vi "Day06-03_지진 계측기.vi"() -> ()   [LabVIEW 2021]
uses:
  <vilib>/Utility/sysdir.llb/System Directory Type.ctl
  <vilib>/DAQmx/configure/timing.llb/DAQmx Timing (Sample Clock).vi
  <vilib>/DAQmx/create/channels.llb/DAQmx Create Channel (AI-Voltage-Basic).vi
  <vilib>/DAQmx/read.llb/DAQmx Read (Analog Wfm 1Chan NSamp).vi
  <vilib>/numeric/Random Number (Range) U64.vi
panel:
  in  "정지":bool
  in  "파일저장":bool
  in  "알람리셋":bool
  in  "감지시작":bool
  out "알림":bool
  out "출력메시지":string
  out "지진센서값출력":dbl(graph)
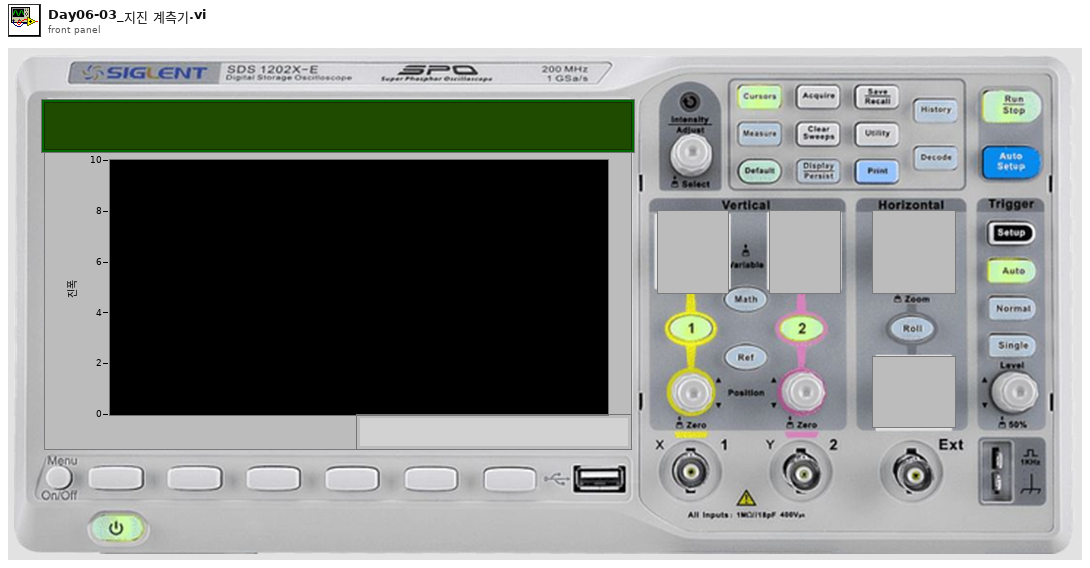
[diagram p1: front panel]
types:
  T1 = typedef "지진 계측기 상태 열거형 상수.ctl" = enum16{"초기화", "대기", "감지 시작", "알림 리셋", "정지"}
  T2 = cluster{"상태":T1, "알림":bool, "출력메시지":string, "지진센서값":dbl, "시간상수":i32}
  T3 = typedef "컨트롤 5.ctl" = enum16{"초기화", "대기", "감지시작", "알람리셋", "정지", "파일저장"}
  T4 = enum16{"open", "replace", "create", "open or create", "replace or create", "replace or create with confirmation"}
  T5 = typedef "System Directory Type.ctl" = i32
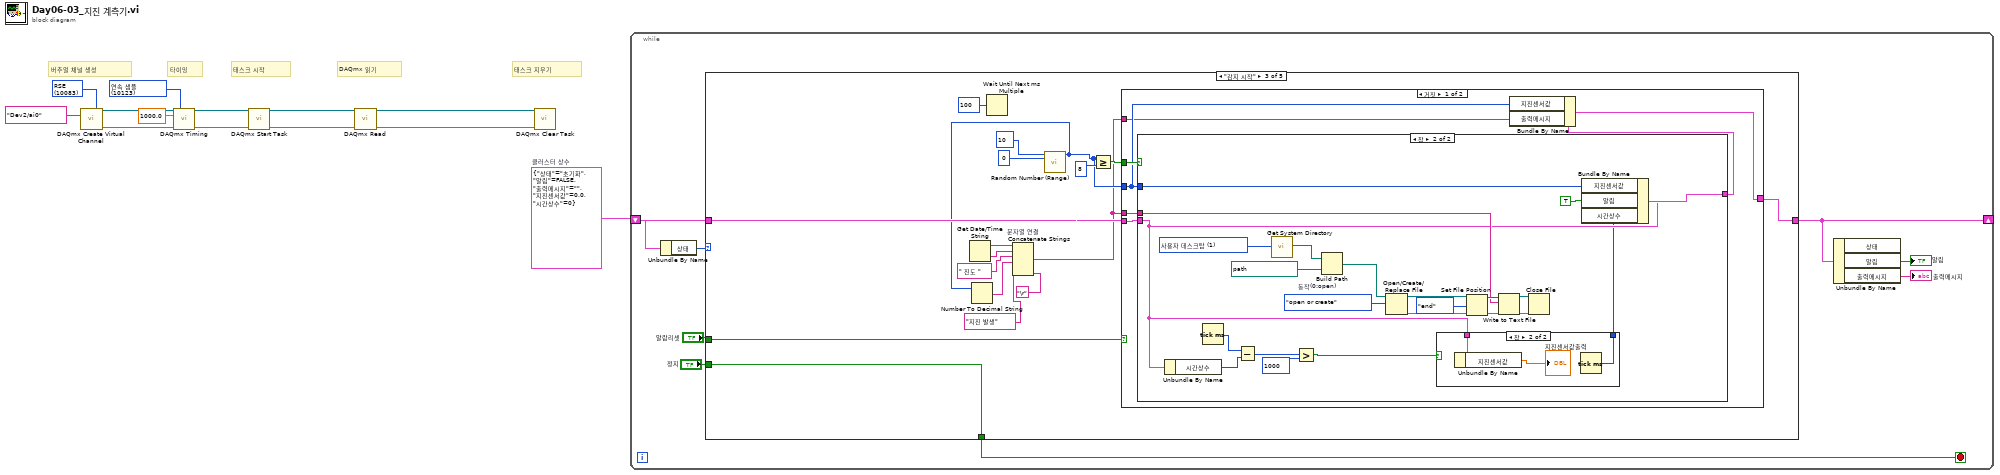
[diagram p0: block diagram]
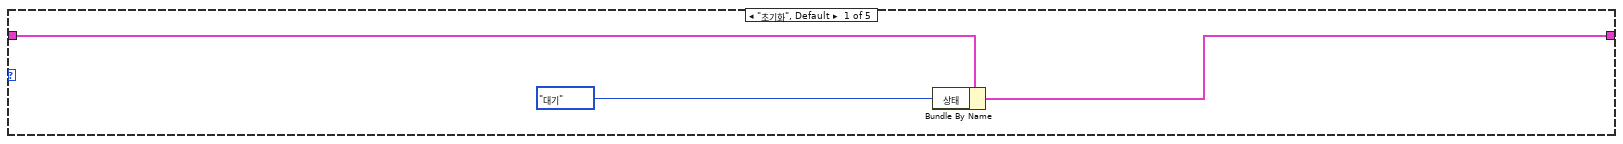
[diagram p2: hidden frame]
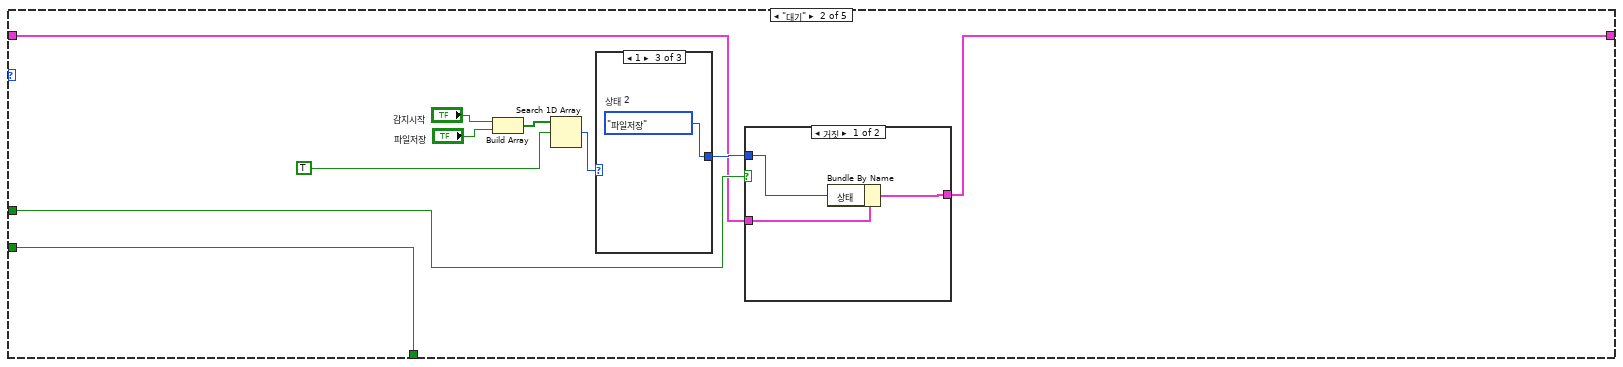
[diagram p3: hidden frame]
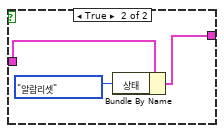
[diagram p4: hidden frame]
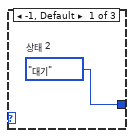
[diagram p5: hidden frame]
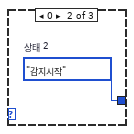
[diagram p6: hidden frame]
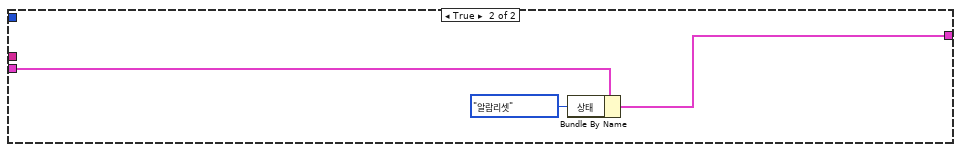
[diagram p9: hidden frame]
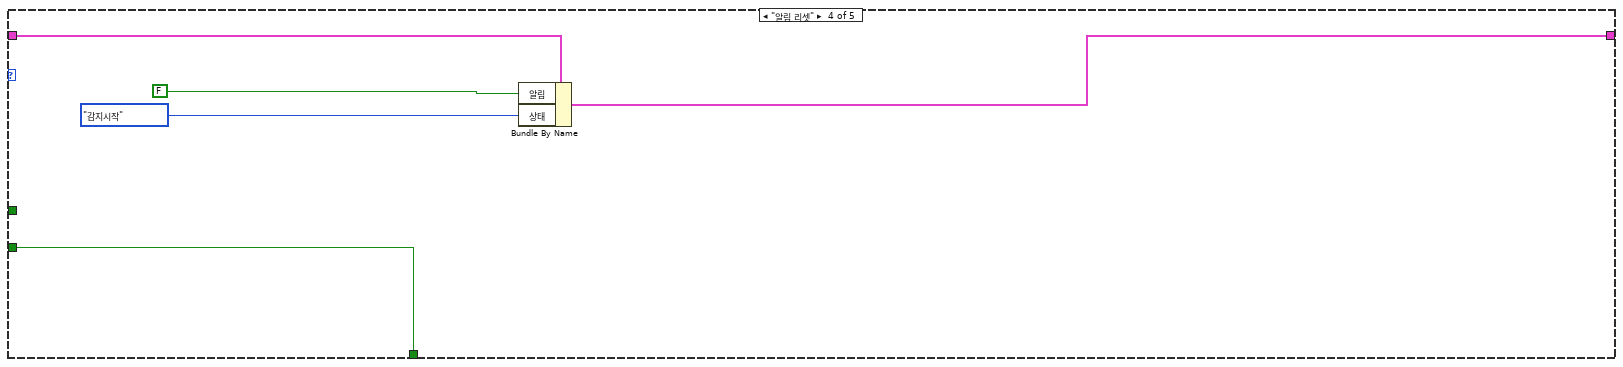
[diagram p10: hidden frame]
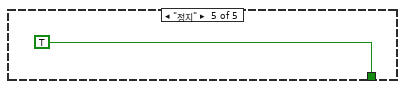
[diagram p11: hidden frame]
diagram:
  w2 = 10123 items=["유한 샘플"=10178, "연속 샘플"=10123, "하드웨어 타이밍에 의한 단일 포인트"=12522] ("sample mode")
  w3 = 10083 items=["기본"=-1, "RSE"=10083, "NRSE"=10078, "차동"=10106, "유사 차동"=12529] ("input terminal configuration")
  w13 = T2 {"상태"=enum."초기화", "알림"=FALSE, "출력메시지"="", "지진센서값"=0.0, "시간상수"=0}  # 클러스터 상수
  # "DAQmx 읽기"
  # "타이밍"
  # "태스크 지우기"
  # "태스크 시작"
  # "버추얼 채널 생성"
  n1 = call-poly <vilib>:"DAQmx Create Virtual Channel.vi"("input terminal configuration"=w3, "physical channels"=tag "Dev2/ai0") -> ("task out"=w12:refnum<k21>, "error out"=w11:errorcluster)  [unwired: 12 in]
  n2 = call-poly <vilib>:"DAQmx Timing.vi"("task/channels in"=w12, "sample mode"=w2, "rate"=1000.0, "error in"=w11) -> ("task out"=w10:refnum<k21>, "error out"=w9:errorcluster)  [unwired: 10 in]
  n3 = call <vilib>:"DAQmx Start Task.vi"("task/channels in"=w10, "error in"=w9) -> ("task out"=w7:refnum<k21>, "error out"=w6:errorcluster)  [unwired: 12 in]
  n4 = call-poly <vilib>:"DAQmx Read.vi"("task/channels in"=w7, "error in"=w6) -> ("task out"=w5:refnum<k21>, "error out"=w4:errorcluster)  [unwired: 11 in, 1 out]
  n5 = call <vilib>:"DAQmx Clear Task.vi"("task in"=w5, "error in"=w4) -> ()  [unwired: 13 in, 1 out]
  n6 = while {
    shift-right: [w20] -> _
    shift-left: w13 -> [w21]
    stop <- w19 stop-if-true
    n7 = Unbundle By Name(w21) -> ("상태"=w14:T1)
    n8 = case shown="\"감지 시작\"" w14 {
      tunnel: [w23 w27 w55 w99 _] -> w20
      tunnel: w21 -> [w24 w25 w54 w102 _]
      tunnel: [_ w26 w44 w98 TRUE] -> w19
      tunnel: "알람리셋" -> [_ w29 w53 _ _]
      tunnel: "정지" -> [_ w26 w44 w98 _]
      frame "초기화", Default {
        n9 = Bundle By Name(cluster=w24, "상태"=지진_계측기_상태_열거형_상수."대기") -> (w23:T2)
      }
      frame "대기" {
        n10 = Build Array("감지시작", "파일저장") -> (w34:bool[])
        n11 = Search 1D Array(1D array=w34, element=TRUE ("원소")) -> (index of element=w32:i32)  [unwired: 1 in]
        n12 = case shown="1" w32 {
          tunnel: [w41 w42 w43] -> w28
          frame -1, Default {
            w41 = 지진_계측기_상태_열거형_상수."대기"  # 상태 2
          }
          frame 0 {
            w42 = 컨트롤_5."감지시작"  # 상태 2
          }
          frame 1 {
            w43 = 컨트롤_5."파일저장"  # 상태 2
          }
        }
        n13 = case shown="거짓" w29 {
          tunnel: w28 -> [w35 _]
          tunnel: [w36 w40] -> w27
          tunnel: w25 -> [w37 w39]
          frame False {
            n14 = Bundle By Name(cluster=w37, "상태"=w35) -> (w36:T2)
          }
          frame True {
            n15 = Bundle By Name(cluster=w39, "상태"=컨트롤_5."알람리셋") -> (w40:T2)
          }
        }
      }
      frame "감지 시작" {
        n16 = Get Date/Time String() -> (date string=w49:string, time string=w48:string)  [unwired: 3 in]
        n17 = Wait Until Next ms Multiple(millisecond multiple=u32 100 ("ms 배수")) -> ()  [unwired: 1 out]
        n18 = call-poly <vilib>:"Random Number (Range).vi"("lower bound (0)"=u64 0, "upper bound (100)"=u64 10) -> ("number"=w46:u64)  [unwired: 9 in]
        n19 = Number To Decimal String(number=w46) -> (decimal integer string=w47:string)  [unwired: 1 in]
        n20 = Concatenate Strings "문자열 연결"(w49, w48, " 진도 " ("문자열"), w47, "지진 발생" ("문자열"), "\r") -> (w45:string)
        n21 = Greater Or Equal?(x=w46, y=u64 8) -> (x >= y?=w56:bool)
        n22 = case shown="거짓" w53 {
          tunnel: w56 -> [w67 _]
          tunnel: [w65 w96] -> w55
          tunnel: w54 -> [w64 w97]
          tunnel: w46 -> [w63 _]
          tunnel: w45 -> [w62 _]
          tunnel: w45 -> [w61 _]
          frame False {
            n23 = case shown="참" w67 {
              tunnel: w64 -> [w68 w70]
              tunnel: w63 -> [_ w91]
              tunnel: [w68 w90] -> w66
              tunnel: w61 -> [_ w77]
              frame False {
              }
              frame True {
                w80 = T4."open or create"  # 동작(0:open)
                w78 = T5 1 items=["사용자 홈"=0, "사용자 데스크탑"=1, "사용자 문서"=2, "사용자 어플리케이션 데이터"=3, "사용자 환경"=4, "사용자 임시"=5, "퍼블릭 문서"=6, "퍼블릭 어플리케이션 데이터"=7, "퍼블릭 환경"=8, "퍼블릭 캐시"=13, "시스템 코어 라이브러리"=9, "시스템 설치된 라이브러리"=10, "어플리케이션 파일"=11, "부팅 볼륨 루트"=12] ("system directory type")
                n24 = Unbundle By Name(w70) -> ("시간상수"=w74:i32)
                n25 = Tick Count (ms)() -> (millisecond timer value=w75:u32)
                n26 = Subtract(x=w75, y=w74) -> (x-y=w73:u32)
                n27 = call <vilib>:"Get System Directory.vi"("system directory type"=w78) -> ("system directory"=w76:path)  [unwired: 10 in]
                n28 = Greater?(x=w73, y=u32 1000) -> (0:w71:bool)
                n29 = Build Path ("경로 만들기")(base path=w76, name or relative path=path "날짜_Log.txt" ("이름 또는 상대 경로")) -> (appended path=w88:path)
                n30 = Open/Create/Replace File ("파일 열기/생성/대체")(file path (use dialog)=w88, operation (0:open)=w80) -> (refnum out=w83:refnum<file>, error out=w82:errorcluster)  [unwired: 4 in, 1 out]
                n31 = case shown="참" w71 {
                  tunnel: w70 -> [_ w94]
                  tunnel: [_ w92] -> w69
                  frame False {
                  }
                  frame True {
                    n32 = Unbundle By Name(w94) -> ("지진센서값"=→"지진센서값출력":dbl)
                    n33 = Tick Count (ms)() -> (millisecond timer value=w92:u32)
                  }
                }
                n34 = Set File Position ("파일 위치 설정")(refnum=w83, from (0:start)=enum16{"start", "end", "current"}."end" ("위치(0:start)"), error in=w82) -> (refnum out=w85:refnum<file>, error out=w84:errorcluster)  [unwired: 1 in]
                n35 = Write to Text File ("텍스트 파일에 쓰기")(file (use dialog)=w85, text=w77, error in=w84) -> (refnum out=w87:refnum<file>, error out=w86:errorcluster)  [unwired: 1 in, 1 out]
                n36 = Close File ("파일 닫기")(refnum=w87, error in=w86) -> ()  [unwired: 2 out]
                n37 = Bundle By Name(cluster=w70, "지진센서값"=w91, "알림"=TRUE, "시간상수"=w69) -> (w90:T2)
              }
            }
            n38 = Bundle By Name(cluster=w66, "지진센서값"=w63, "출력메시지"=w62) -> (w65:T2)
          }
          frame True {
            n39 = Bundle By Name(cluster=w97, "상태"=컨트롤_5."알람리셋") -> (w96:T2)
          }
        }
      }
      frame "알림 리셋" {
        n40 = Bundle By Name(cluster=w102, "알림"=FALSE, "상태"=컨트롤_5."감지시작") -> (w99:T2)
      }
      frame "정지" {
      }
    }
    n41 = Unbundle By Name(w20) -> ("알림"=→"알림":bool, "출력메시지"=→"출력메시지":string)  [unwired: 1 out]
  }
